vi "Wrapper_setIntegrationTime.vi"(1 "Integration Time":i32, 2 "Index":i32, 3 "Wrapper In":u32) -> (0 "Wrapper Out":u32)   [LabVIEW 2017]
uses:
  OmniDriver32.dll
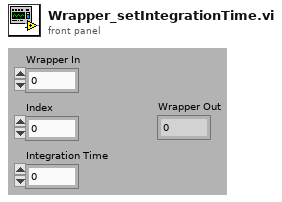
[diagram p1: front panel]
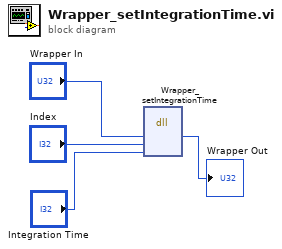
[diagram p0: block diagram]
diagram:
  n1 = dll-call lib="OmniDriver32.dll" fn="Wrapper_setIntegrationTime" label="Wrapper.setIntegrationTime"("Wrapper"="Wrapper In", "Index"="Index", "Integration Time"="Integration Time") -> ("Wrapper"=→"Wrapper Out":u32)  [unwired: 5 in, 3 out]
